vi "Test_IR_Range_Finder.vi"() -> ()   [LabVIEW 2011]
panel:
  out "Average Distance (in)\nOver 10 Readings":dbl
  out "Distance (in) Graph":dbl(graph)
  out "Instantaneous Distance (in)":dbl
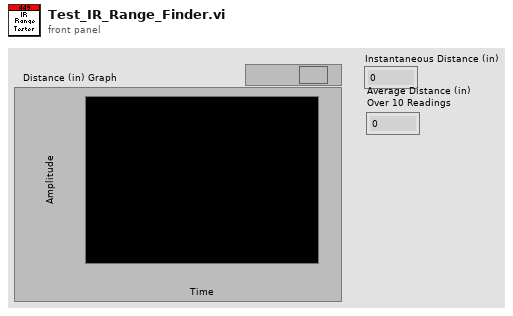
[diagram p1: front panel]
types:
  T1 = typedef "WPI_AnalogChannelDevRef.ctl" = cluster{"DevStatus":errorcluster, "Analog Module":T2, "Analog Channel":T3}
  T2 = typedef "FPGA_TypedefAnalogModule.ctl" = enum16{"Analog Module 1", "Analog Module 2"}
  T3 = typedef "FPGA_AIChannel.ctl" = enum8{"AI 1", "AI 2", "AI 3", "AI 4", "AI 5", "AI 6", "AI 7", "AI 8", "Invalid"}
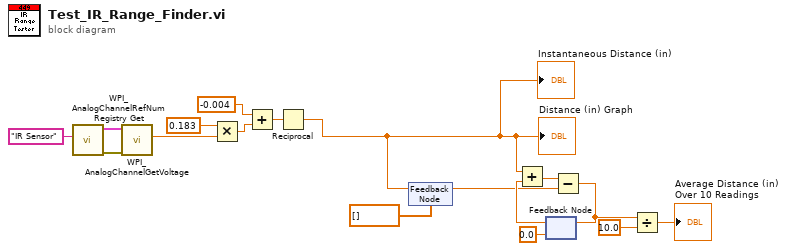
[diagram p0: block diagram]
diagram:
  n1 = call <vilib>:"WPI_AnalogChannelRefNum Registry Get.vi"("refnum name"="IR Sensor") -> ("error out"=w16:errorcluster, "AIDeviceRef"=w15:T1)  [unwired: 9 in]
  n2 = call <vilib>:"WPI_AnalogChannelGetVoltage.vi"("error in (no error)"=w16, "AIDeviceRef"=w15) -> ("Voltage"=w4:dbl)  [unwired: 7 in, 2 out]
  n3 = Multiply(x=0.183, y=w4) -> (x*y=w6:dbl)
  n4 = Add(x=-0.004, y=w6) -> (x+y=w5:dbl)
  n5 = Reciprocal(x=w5) -> (1/x=w3:dbl)
  "Instantaneous Distance (in)" <- w3
  "Distance (in) Graph" <- w3
  n6 = feedback-in #1(w3) -> ()
  n7 = feedback #1(dbl[] []) -> (w12:dbl)
  n8 = feedback #2(0.0) -> (w14:dbl)
  n9 = Add(x=w3, y=w14) -> (x+y=w13:dbl)
  n10 = Subtract(x=w13, y=w12) -> (x-y=w9:dbl)
  n11 = feedback-in #2(w9) -> ()
  n12 = Divide(x=w9, y=10.0) -> (x/y=→"Average Distance (in)\nOver 10 Readings":dbl)
